vi "Dialogue_Error.vi"(8 "error in":errorcluster) -> (0 "error out":errorcluster)   [LabVIEW 2014, in "hse-ui.lvlib"]
doc: "Shows a dialog window for displaying an error message.\n\n____\nHAMPEL SOFTWARE ENGINEERING v0.7.0 (2018-07-16 18:12)"
uses:
  hse-ui.lvlib
  FPControl/FPControl_Actions.ctl
panel:
  out "Message":string caption="Enter Application Name"
  in  "Btn_OK":bool
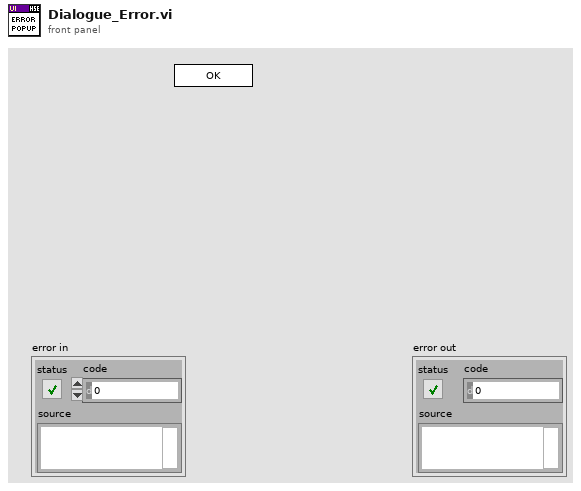
[diagram p1: front panel]
types:
  T1 = typedef "hse-ui.lvlib/FPControl_Actions.ctl" = enum16{"Open", "Hide", "Close", "Bring To Front", "Center", "Minimize", "Maximize"}
  T2 = typedef "LVRectTypeDef.ctl" = cluster{"Left":i16, "Top":i16, "Right":i16, "Bottom":i16}
  T3 = cluster{"left":i16, "top":i16, "right":i16, "bottom":i16}
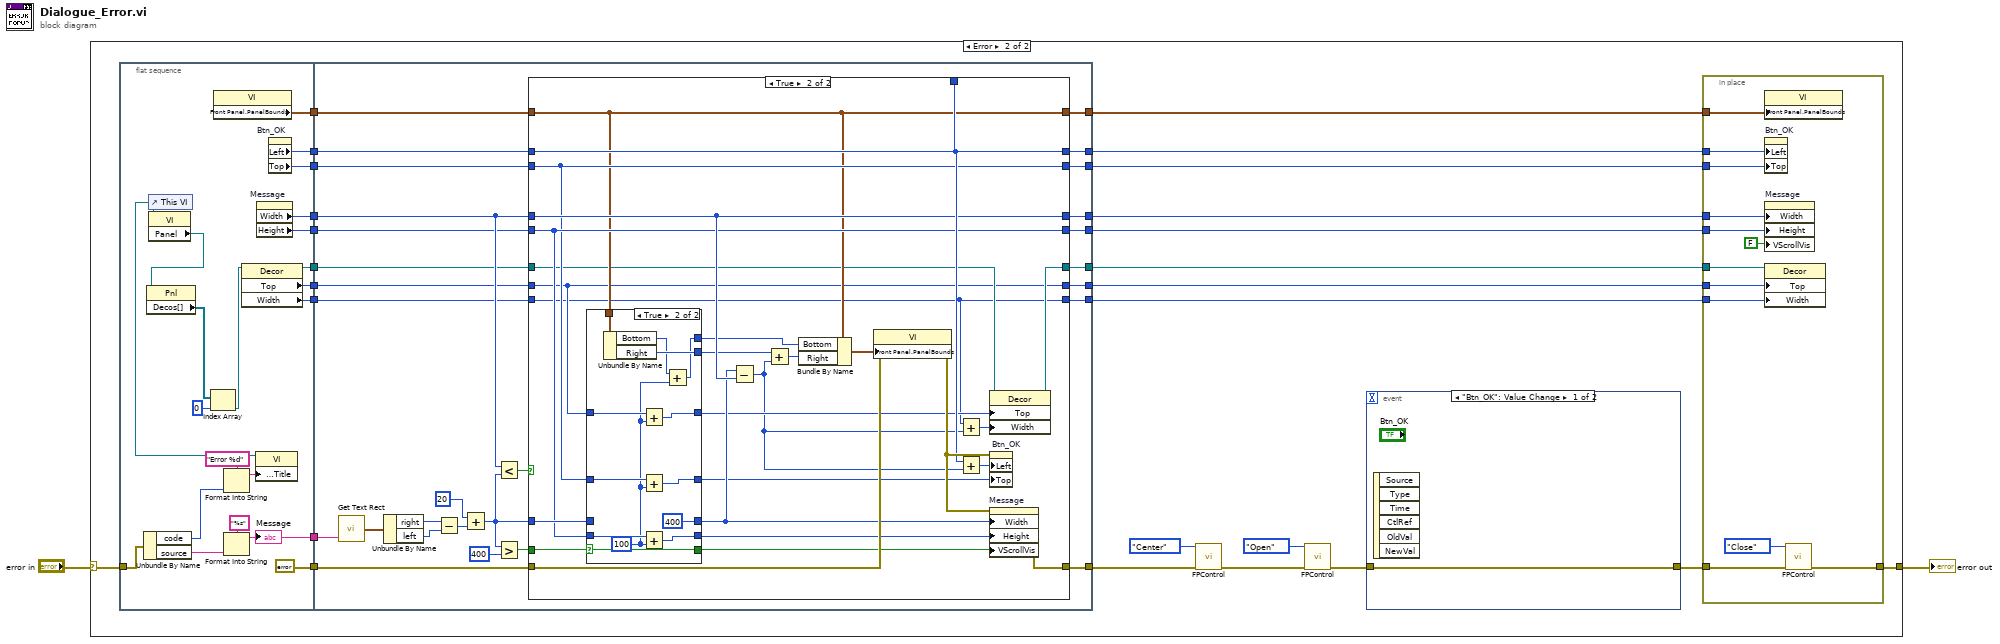
[diagram p0: block diagram]
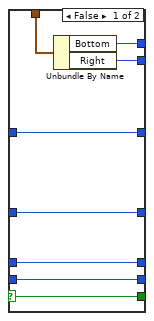
[diagram p4: hidden frame]
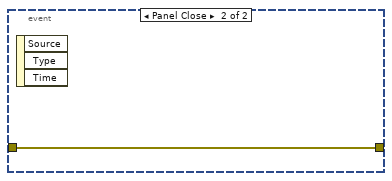
[diagram p5: hidden frame]
diagram:
  n1 = case shown="Error" "error in" {
    selector: "error in" -> [w3 w23]
    tunnel: [w3 w26] -> w2
    frame No Error {
    }
    frame Error {
      n2 = flat-sequence {
        tunnel: w23 -> [w50]
        tunnel: [w44] -> w19
        tunnel: [w43] -> w18
        tunnel: [w42] -> w17
        tunnel: [w41] -> w16
        tunnel: [errorcluster {"status"=FALSE, "code"=0, "source"=""} ("error in")] -> w15
        tunnel: [w39] -> w14
        tunnel: [w38] -> w11
        tunnel: [w36] -> w9
        tunnel: [w31] -> w8
        tunnel: [w30] -> w6
        tunnel: [w66] -> w21
        tunnel: [w68] -> w20
        tunnel: w19 -> [w63]
        tunnel: w18 -> [w69]
        tunnel: w17 -> [w67]
        tunnel: [w70] -> w22
        tunnel: w16 -> [w72]
        tunnel: w15 -> [w71]
        tunnel: w14 -> [w65]
        tunnel: [w64] -> w13
        tunnel: [w61] -> w12
        tunnel: w11 -> [w60]
        tunnel: [w62] -> w10
        tunnel: w9 -> [w56]
        tunnel: w8 -> [w55]
        tunnel: [w54] -> w7
        tunnel: w6 -> [w53]
        tunnel: [w52] -> w5
        tunnel: [w51] -> w4
        frame #0 {
          n3 = Unbundle By Name(w50) -> ("code"=w46:i32, "source"=w47:string)
          n4 = control-ref of="This VI"() -> (w37:refnum<vi>)
          n5 = property class="VI"(reference=w37) -> ("Panel"=w32:refnum<vi>)  [unwired: 1 in, 2 out]
          n6 = property class="Pnl"(reference=w32) -> ("Decos[]"=w34:refnum<vi>[])  [unwired: 1 in, 2 out]
          n7 = Index Array(array=w34, index=0) -> (element=w35:refnum<vi>)
          n8 = property class="VI"() -> ("Front Panel.PanelBounds"=w43:T2)  [unwired: 2 in, 2 out]
          n9 = Format Into String(format string="Error %d", w46) -> (resulting string=w49:string)  [unwired: 2 in, 1 out]
          n10 = Format Into String(format string="%s", w47) -> (resulting string=w41:string)  [unwired: 2 in, 1 out]
          "Message" <- w41
          n11 = property class="Decor"(reference=w35) -> (reference out=w31:refnum<vi>, "Top"=w36:i32, "Width"=w30:u32)  [unwired: 1 in, 1 out]
          n12 = property class="VI"(reference=w37, "Front Panel.Title"=w49) -> ()  [unwired: 1 in, 2 out]
          n13 = property on="Message" class="Str"() -> ("Width"=w44:u32, "Height"=w38:u32)  [unwired: 2 in, 2 out]
          n14 = property on="Btn_OK" class="Bool"() -> ("Left"=w42:i32, "Top"=w39:i32)  [unwired: 2 in, 2 out]
        }
        frame #1 {
          n15 = call <vilib>:"Get Text Rect.vi"("text"=w72) -> ("rect"=w73:T3)  [unwired: 8 in]
          n16 = Unbundle By Name(w73) -> ("right"=w74:i16, "left"=w75:i16)
          n17 = Subtract(x=w74, y=w75) -> (x-y=w77:i16)
          n18 = Add(x=i16 20 ("y"), y=w77) -> (x+y=w58:i16)
          n19 = Less?(x=w63, y=w58) -> (x < y?=w76:bool)
          n20 = Greater?(x=w58, y=i16 400) -> (0:w57:bool)
          n21 = case shown="True" w76 {
            tunnel: w58 -> [_ w105]
            tunnel: w71 -> [w87 w110]
            tunnel: [w87 w95] -> w70
            tunnel: w67 -> [_ _]
            tunnel: w69 -> [w86 w98]
            tunnel: [w86 w98] -> w68
            tunnel: w67 -> [w85 w108]
            tunnel: [w85 w108] -> w66
            tunnel: w65 -> [w84 w100]
            tunnel: [w84 w100] -> w64
            tunnel: w63 -> [w83 w107]
            tunnel: [w83 w107] -> w62
            tunnel: [w82 w101] -> w61
            tunnel: w60 -> [w82 w101]
            tunnel: w57 -> [_ w106]
            tunnel: w56 -> [w80 w91]
            tunnel: w55 -> [w81 w93]
            tunnel: [w81 w92] -> w54
            tunnel: w53 -> [w79 w89]
            tunnel: [w80 w91] -> w52
            tunnel: [w79 w89] -> w51
            frame False {
            }
            frame True {
              n22 = case shown="True" w106 {
                selector: w106 -> [w119 w134]
                tunnel: w105 -> [w120 _]
                tunnel: [w120 i16 400] -> w104
                tunnel: [w119 w134] -> w103
                tunnel: [w121 w131] -> w102
                tunnel: w101 -> [w121 w133]
                tunnel: w100 -> [w118 w127]
                tunnel: [w118 w128] -> w99
                tunnel: w98 -> [w115 w129]
                tunnel: [w117 w130] -> w97
                tunnel: [w116 w125] -> w96
                tunnel: [w114 w122] -> w94
                tunnel: w91 -> [w114 w124]
                frame False {
                  n23 = Unbundle By Name(w115) -> ("Bottom"=w116:i16, "Right"=w117:i16)
                }
                frame True {
                  w123 = u32 100 ("y")
                  n24 = Unbundle By Name(w129) -> ("Bottom"=w126:i16, "Right"=w130:i16)
                  n25 = Add(x=w124, y=w123) -> (x+y=w122:u32)
                  n26 = Add(x=w127, y=w123) -> (x+y=w128:u32)
                  n27 = Add(x=w133, y=w123) -> (x+y=w131:u32)
                  n28 = Add(x=w126, y=w123) -> (x+y=w125:u32)
                }
              }
              n29 = Subtract(x=w104, y=w107) -> (x-y=w88:u32)
              n30 = Add(x=w97, y=w88) -> (x+y=w113:u32)
              n31 = Bundle By Name(cluster=w98, "Bottom"=w96, "Right"=w113) -> (w112:T2)
              n32 = property class="VI"(error in=w110, "Front Panel.PanelBounds"=w112) -> (error out=w111:errorcluster)  [unwired: 1 in, 1 out]
              n33 = Add(x=w89, y=w88) -> (x+y=w90:u32)
              n34 = Add(x=w108, y=w88) -> (x+y=w109:u32)
              n35 = property class="Decor"(reference=w93, "Top"=w94, "Width"=w90) -> (reference out=w92:refnum<vi>)  [unwired: 1 in, 1 out]
              n36 = property on="Message" class="Str"(error in=w111, "Width"=w104, "Height"=w102, "VScrollVis"=w103) -> (error out=w95:errorcluster)  [unwired: 1 in, 1 out]
              n37 = property on="Btn_OK" class="Bool"(error in=w111, "Left"=w109, "Top"=w99) -> ()  [unwired: 1 in, 2 out]
            }
          }
        }
      }
      n38 = call "FPControl.vi"("error in"=w22, "Function"=FPControl_Actions."Center") -> ("error out"=w27:errorcluster)  [unwired: 9 out]
      n39 = call "FPControl.vi"("error in"=w27, "Function"=FPControl_Actions."Open") -> ("error out"=w24:errorcluster)  [unwired: 9 out]
      n40 = event shown="[0] \"Btn_OK\": Value Change" {
        selector: _ -> [_ _]
        dyn-events: _ -> [_ _]
        timeout: _ -> [_ _]
        tunnel: w24 -> [w147 w148]
        tunnel: [w147 w148] -> w25
        event "Btn_OK": Value Change {
          n41 = event-data() -> ()  [unwired: 1 in, 6 out]
        }
        event Panel Close {
          n42 = event-data() -> ()  [unwired: 1 in, 3 out]
        }
      }
      n43 = in-place {
        in-place-border: [w144] -> w26
        in-place-border: w25 -> [w145]
        in-place-border: w21 -> [w143]
        in-place-border: w20 -> [w142]
        in-place-border: w10 -> [w141]
        in-place-border: w13 -> [w139]
        in-place-border: w12 -> [w138]
        in-place-border: w7 -> [w137]
        in-place-border: w5 -> [w136]
        in-place-border: w4 -> [w135]
        n44 = property class="VI"("Front Panel.PanelBounds"=w142) -> ()  [unwired: 2 in, 2 out]
        n45 = property on="Btn_OK" class="Bool"("Left"=w143, "Top"=w139) -> ()  [unwired: 2 in, 2 out]
        n46 = property on="Message" class="Str"("Width"=w141, "Height"=w138, "VScrollVis"=FALSE ("Vertical Scrollbar Visible")) -> ()  [unwired: 2 in, 2 out]
        n47 = property class="Decor"(reference=w137, "Top"=w136, "Width"=w135) -> ()  [unwired: 1 in, 2 out]
        n48 = call "FPControl.vi"("error in"=w145, "Function"=FPControl_Actions."Close") -> ("error out"=w144:errorcluster)  [unwired: 9 out]
      }
    }
  }
  "error out" <- w2
